vi "RotationSpeedSet.vi"(3 "error in (no error)":errorcluster, 4 "Rotation Speed":u16=1 min=1 step=1, 5 "VISA resource name":refnum<visa-resource-name>) -> (0 "error out":errorcluster, 1 "Command not accepted":bool, 2 "VISA resource name out":refnum<visa-resource-name>)   [LabVIEW 2017, in "Spectral Products CM110.lvlib"]
uses:
  Spectral Products CM110.lvlib
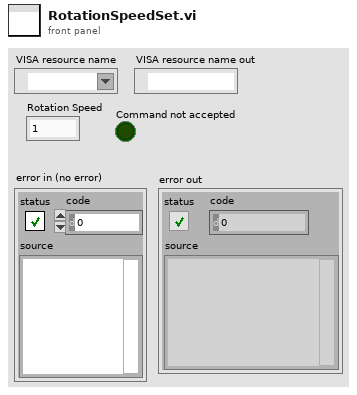
[diagram p1: front panel]
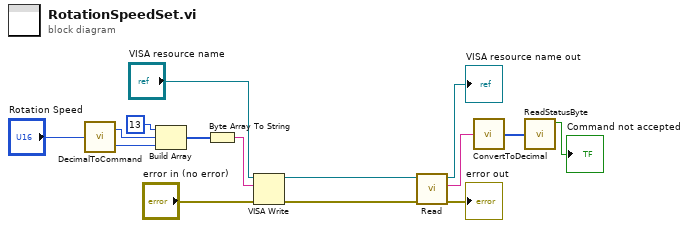
[diagram p0: block diagram]
diagram:
  n1 = call "DecimalToCommand.vi"("Decimal"="Rotation Speed") -> ("HiByte"=w6:u8, "LoByte"=w5:u8)  [unwired: 4 in]
  n2 = Build Array(u8 13, w6, w5) -> (w4:u8[])
  n3 = Byte Array To String(unsigned byte array=w4) -> (string=w3:string)
  n4 = VISA Write(VISA resource name="VISA resource name", write buffer=w3, error in (no error)="error in (no error)") -> (VISA resource name out=w2:refnum<visa-resource-name>, error out=w1:errorcluster)  [unwired: 1 out]
  n5 = call "Read.vi"("error in (no error)"=w1, "VISA Refnum in"=w2) -> ("error out"=→"error out":errorcluster, "read buffer"=w11:string, "VISA Refnum out"=→"VISA resource name out":refnum<visa-resource-name>)  [unwired: 6 in, 1 out]
  n6 = call "ConvertToDecimal.vi"("read buffer"=w11) -> ("unsigned byte array"=w10:u8[])
  n7 = call "ReadStatusByte.vi"("unsigned byte array"=w10) -> ("Command not accepted"=→"Command not accepted":bool)  [unwired: 4 in, 5 out]
